vi "Init LED page.vi"(7 "Card Position":refnum<vi>, 8 "error in (no error)":errorcluster, 9 "Description":refnum<vi>, 10 "Name":refnum<vi>, 11 "Node Ptr":T2 format="%.0x") -> (0 "error out":errorcluster, 2 "LED States":T1[](array[typedef]), 3 "Node Ptr out":T2 format="%.0x")   [LabVIEW 2014, in "SLSC configuration System Explorer.lvlib"]
uses:
  SLSC configuration System Explorer.lvlib
  <vilib>/NI Veristand/Custom Device API/Custom Device Item Ref.ctl
  Shared/LED Backplane/LED State.ctl
  <vilib>/NI Veristand/Custom Device API/Custom Device API.lvlib
  Shared/SLSC configuration Shared.lvlib
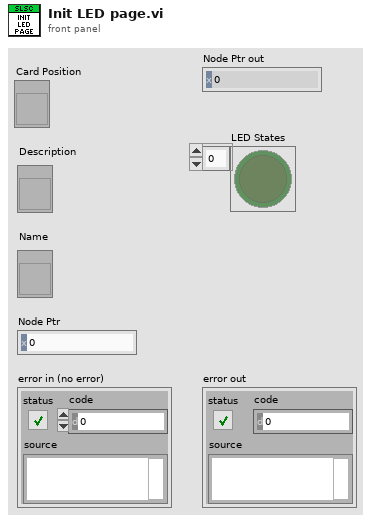
[diagram p1: front panel]
types:
  T1 = typedef "SLSC configuration Shared.lvlib/LED State.ctl" = bool
  T2 = typedef "Custom Device API.lvlib/Custom Device Item Ref.ctl" = u64
  T3 = typedef "Custom Device API.lvlib/Custom Device Item Info.ctl" = cluster{"Name":string, "Is Channel":bool, "GUID":string, "Is Waveform":bool}
  T4 = typedef "SLSC configuration Shared.lvlib/Card Position.ctl" = cluster{"Rack #":u8, "Slot #":T5}
  T5 = typedef "SLSC configuration Shared.lvlib/Slot #.ctl" = u8
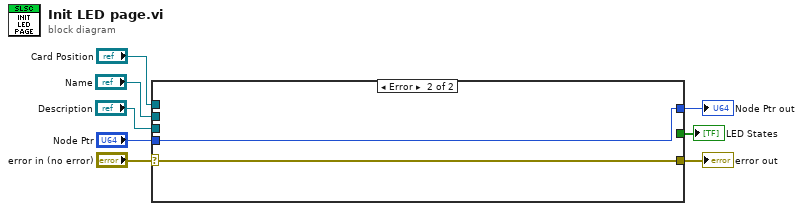
[diagram p0: block diagram]
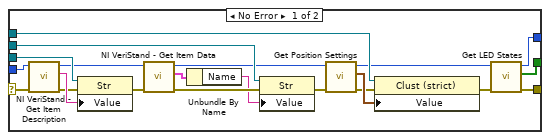
[diagram p2: hidden frame]
diagram:
  n1 = case shown="Error" "error in (no error)" {
    selector: "error in (no error)" -> [w17 w31]
    tunnel: "Name" -> [w29 _]
    tunnel: "Description" -> [w25 _]
    tunnel: [w21 w31] -> w6
    tunnel: "Node Ptr" -> [w20 w30]
    tunnel: "Card Position" -> [w15 _]
    tunnel: [w10 w30] -> w2
    tunnel: [w9 _] -> w1
    frame No Error {
      n2 = call <vilib>:"NI VeriStand - Get Item Description.vi"("error in (no error)"=w17, "Item Ref in"=w20) -> ("error out"=w24:errorcluster, "Description"=w26:string, "Item Ref out"=w22:T2)  [unwired: 7 out]
      n3 = property class="Str"(reference=w25, error in=w24, "Value"=w26) -> (error out=w27:errorcluster)  [unwired: 1 out]
      n4 = call <vilib>:"NI VeriStand - Get Item Data.vi"("error in (no error)"=w27, "Item Ref in"=w22) -> ("error out"=w28:errorcluster, "Item Info"=w23:T3, "Item Ref out"=w18:T2)  [unwired: 7 out]
      n5 = Unbundle By Name(w23) -> ("Name"=w14:string)
      n6 = property class="Str"(reference=w29, error in=w28, "Value"=w14) -> (error out=w19:errorcluster)  [unwired: 1 out]
      n7 = call "Get Position Settings.vi"("error in (no error)"=w19, "Item Ref in"=w18) -> ("error out"=w11:errorcluster, "Card Position"=w13:T4, "Item Ref out"=w12:T2)  [unwired: 7 in]
      n8 = property class="Clust (strict)"(reference=w15, error in=w11, "Value"=w13) -> (error out=w16:errorcluster)  [unwired: 1 out]
      n9 = call "Get LED States.vi"("error in (no error)"=w16, "LED Board Ref in"=w12) -> ("error out"=w21:errorcluster, "LED States"=w9:T1[], "LED Board Ref out"=w10:T2)  [unwired: 6 in, 1 out]
    }
    frame Error {
    }
  }
  "Node Ptr out" <- w2
  "error out" <- w6
  "LED States" <- w1
